vi "Set_Det.vi"(8 "error in (no error)":errorcluster, 11 "Control-Server in":refnum<class "Control-Server.lvclass">) -> (0 "error out":errorcluster, 3 "Control-Server out":refnum<class "Control-Server.lvclass">)   [LabVIEW 2020, in "Control-Server.lvclass"]
uses:
  Control-Server.lvclass
  Config/config_names_def.ctl
  Detector/Emulate/Emulate.lvclass
  C:/Dev/TRANCON/Classes/Detector/Detector.lvclass
  Detector/VIS-IR/VIS-NIR.lvclass
  Detector/UV-VIS/CCD_camera.lvclass
  Detector/DET_BUNCH/Avantes_bunch.lvclass
  Detector/UV-VIS_AVANTES/UV-VIS_AVANTES.lvclass
  dependecies/ControlsVIs/Clusters-def/Message types.ctl
  Message/Message.lvclass
  Message/Message.lvclass/Message.ctl
  GeneralFunctionality/GeneralFunctionality.lvclass/GeneralFunctionality.ctl
  Detector/Detector.lvclass/Detector.ctl
  Control-Server.lvclass/Control-Server.ctl
  Detector/Detector.lvclass
  C:/Dev/TRANCON/Classes/GeneralFunctionality/GeneralFunctionality.lvclass
  Config/Config.lvclass
  GeneralFunctionality/GeneralFunctionality.lvclass
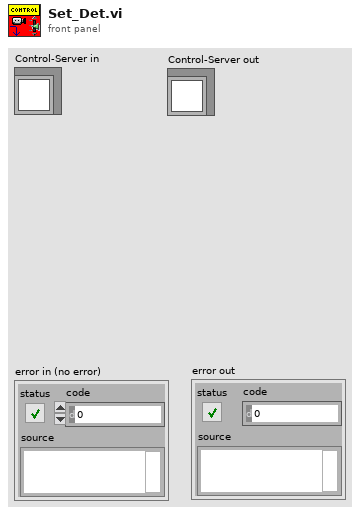
[diagram p1: front panel]
types:
  T1 = typedef "Message types.ctl" = string
  T2 = typedef "Config.lvclass/config_names_def.ctl" = string
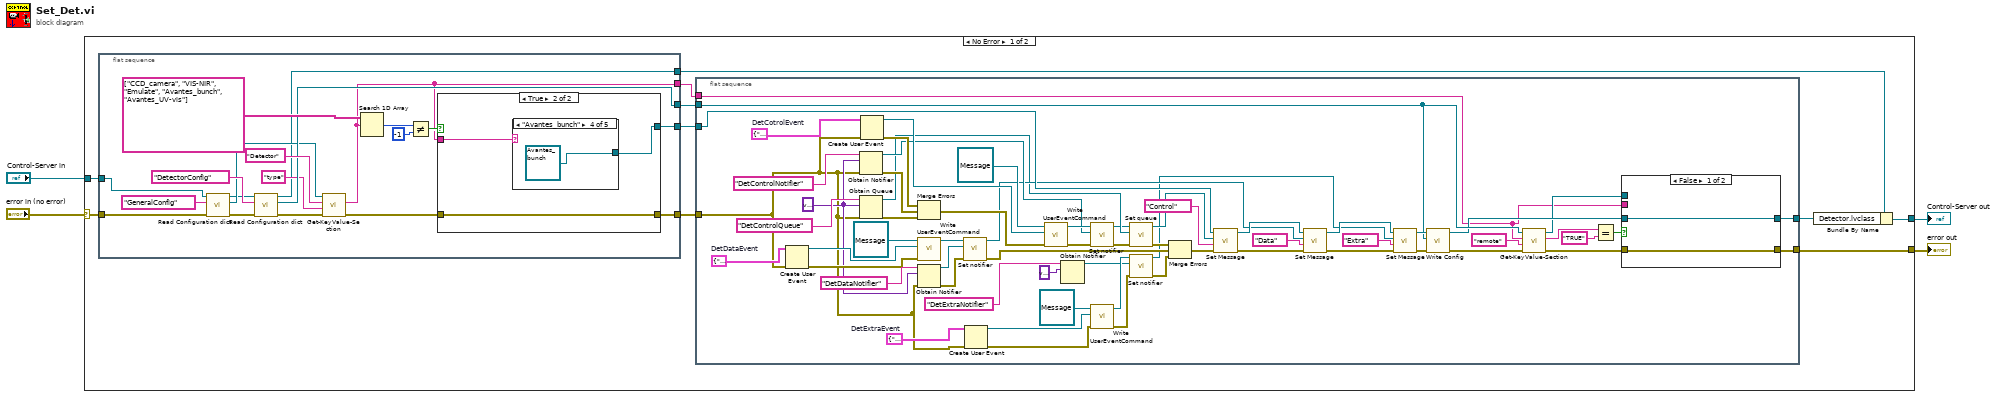
[diagram p0: block diagram]
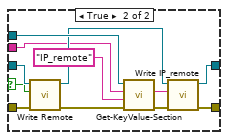
[diagram p2: hidden frame]
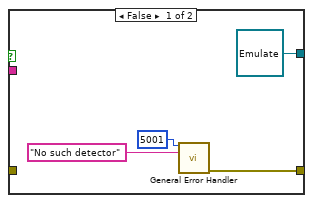
[diagram p3: hidden frame]
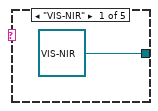
[diagram p4: hidden frame]
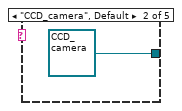
[diagram p5: hidden frame]
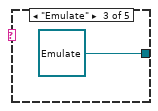
[diagram p6: hidden frame]
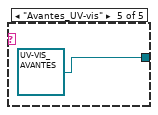
[diagram p7: hidden frame]
diagram:
  n1 = case shown="No Error" "error in (no error)" {
    selector: "error in (no error)" -> [w8 w124]
    tunnel: [w11 w125] -> w4
    tunnel: "Control-Server in" -> [w10 w125]
    tunnel: [w6 w124] -> w2
    frame No Error {
      n2 = flat-sequence {
        tunnel: w10 -> [w101]
        tunnel: w8 -> [w100]
        tunnel: [w103] -> w12
        tunnel: [w93] -> w13
        tunnel: [w102] -> w14
        tunnel: [w94] -> w9
        tunnel: [w92] -> w5
        frame #0 {
          n3 = call "Read Configuration dict.vi"("error in (no error)"=w100, "Config Name"=T2 "GeneralConfig", "Control in"=w101) -> ("error out"=w97:errorcluster, "Config"=w98:refnum<class "Config.lvclass">, "Control out"=w95:refnum<class "Control-Server.lvclass">)  [unwired: 6 in]
          n4 = call "Read Configuration dict.vi"("error in (no error)"=w97, "Config Name"=T2 "DetectorConfig", "Control in"=w95) -> ("error out"=w96:errorcluster, "Config"=w103:refnum<class "Config.lvclass">, "Control out"=w94:refnum<class "Control-Server.lvclass">)  [unwired: 6 in]
          n5 = call-dynamic "Get-KeyValue-Section.vi"("error in (no error)"=w96, "Key"="type", "Section"="Detector", "Config in"=w98) -> ("error out"=w105:errorcluster, "Value"=w92:string)  [unwired: 5 in, 1 out]
          n6 = Search 1D Array(1D array=string[] ["CCD_camera", "VIS-NIR", "Emulate", "Avantes_bunch", "Avantes_UV-vis"], element=w92) -> (index of element=w108:i32)  [unwired: 1 in]
          n7 = Not Equal?(x=w108, y=-1) -> (x != y?=w106:bool)
          n8 = case shown="True" w106 {
            tunnel: w92 -> [_ w118]
            tunnel: [refnum<class "Emulate.lvclass"> refnum ("Emulate.lvclass") w116] -> w102
            tunnel: w105 -> [_ w117]
            tunnel: [w113 w117] -> w93
            frame False {
              n9 = call <vilib>:"General Error Handler.vi"("[error code] (0)"=5001 ("code"), "[error source] (\" \")"="No such detector" ("String to Prepend to source (\"\")")) -> ("error out"=w113:errorcluster)  [unwired: 9 in, 4 out]
            }
            frame True {
              n10 = case shown="\"Avantes_bunch\"" w118 {
                tunnel: [refnum<class "VIS-NIR.lvclass"> refnum ("VIS-IR.lvclass") refnum<class "CCD_camera.lvclass"> refnum ("UV-VIS.lvclass") refnum<class "Emulate.lvclass"> refnum ("DETEmulate.lvclass") refnum<class "Avantes_bunch.lvclass"> refnum ("DET_BUNCH.lvclass") refnum<class "UV-VIS_AVANTES.lvclass"> refnum ("UV-VIS_AVANTES.lvclass")] -> w116
                frame "VIS-NIR" {
                }
                frame "CCD_camera", Default {
                }
                frame "Emulate" {
                }
                frame "Avantes_bunch" {
                }
                frame "Avantes_UV-vis" {
                }
              }
            }
          }
        }
      }
      n11 = flat-sequence {
        tunnel: w12 -> [w25]
        tunnel: w13 -> [w34]
        tunnel: w14 -> [w67]
        tunnel: [w24] -> w7
        tunnel: [w23] -> w6
        tunnel: w5 -> [w18]
        frame #0 {
          w35 = cluster{"command":string, "data":variant} {"command"="", "data"=variant}  # DetExtraEvent
          w44 = variant
          w66 = cluster{"command":string, "data":variant} {"command"="", "data"=variant}  # DetDataEvent
          w73 = cluster{"command":string, "data":variant} {"command"="", "data"=variant}  # DetCotrolEvent
          n12 = Create User Event(user event datatype=w66, error in=w34) -> (user event=w62:refnum<user-event>, error out=w61:errorcluster)
          n13 = Obtain Notifier(name (unnamed)="DetControlNotifier" ("nom (aucun)"), notification data type=w44, error in (no error)=w34) -> (notifier out=w69:refnum<notifier>, error out=w70:errorcluster)  [unwired: 1 in, 1 out]
          n14 = Obtain Queue(name (unnamed)="DetControlQueue", element data type=w44, error in (no error)=w34) -> (queue out=w50:refnum<queue>, error out=w49:errorcluster)  [unwired: 2 in, 1 out]
          n15 = Create User Event(user event datatype=w73, error in=w34) -> (user event=w75:refnum<user-event>, error out=w71:errorcluster)
          n16 = Merge Errors(w71, w70, w49) -> (w68:errorcluster)
          n17 = call "Write UserEventCommand.vi"("error in (no error)"=w61, "UserEventCommand"=w62, "Message en entrée"=refnum<class "Message.lvclass"> refnum ("Message.lvclass")) -> ("Message en sortie"=w63:refnum<class "Message.lvclass">)  [unwired: 7 in, 1 out]
          n18 = Obtain Notifier(name (unnamed)="DetDataNotifier" ("nom (aucun)"), notification data type=w44, error in (no error)=w34) -> (notifier out=w59:refnum<notifier>, error out=w60:errorcluster)  [unwired: 1 in, 1 out]
          n19 = call "Set notifier.vi"("error in (no error)"=w60, "notifier"=w59, "Message en entrée"=w63) -> ("error out"=w58:errorcluster, "Message en sortie"=w54:refnum<class "Message.lvclass">)  [unwired: 7 in]
          n20 = Create User Event(user event datatype=w35, error in=w34) -> (user event=w37:refnum<user-event>, error out=w36:errorcluster)
          n21 = call "Write UserEventCommand.vi"("error in (no error)"=w68, "UserEventCommand"=w75, "Message en entrée"=refnum<class "Message.lvclass"> refnum ("Message.lvclass")) -> ("error out"=w72:errorcluster, "Message en sortie"=w76:refnum<class "Message.lvclass">)  [unwired: 7 in]
          n22 = Obtain Notifier(name (unnamed)="DetExtraNotifier" ("nom (aucun)"), notification data type=variant) -> (notifier out=w29:refnum<notifier>)  [unwired: 2 in, 2 out]
          n23 = call "Set notifier.vi"("error in (no error)"=w72, "notifier"=w69, "Message en entrée"=w76) -> ("error out"=w48:errorcluster, "Message en sortie"=w46:refnum<class "Message.lvclass">)  [unwired: 7 in]
          n24 = call "Write UserEventCommand.vi"("error in (no error)"=w36, "UserEventCommand"=w37, "Message en entrée"=refnum<class "Message.lvclass"> refnum ("Message.lvclass")) -> ("error out"=w32:errorcluster, "Message en sortie"=w33:refnum<class "Message.lvclass">)  [unwired: 7 in]
          n25 = call "Set queue.vi"("error in (no error)"=w48, "queue"=w50, "Message in"=w46) -> ("error out"=w47:errorcluster, "Message out"=w45:refnum<class "Message.lvclass">)  [unwired: 7 in]
          n26 = call "Set notifier.vi"("error in (no error)"=w32, "notifier"=w29, "Message en entrée"=w33) -> ("error out"=w28:errorcluster, "Message en sortie"=w39:refnum<class "Message.lvclass">)  [unwired: 7 in]
          n27 = Merge Errors(w47, w58, w28) -> (w57:errorcluster)
          n28 = call "Set Message.vi"("error in (no error)"=w57, "Message type"=T1 "Control", "Message.lvclass"=w45, "GeneralFunctionality en entrée"=w67) -> ("error out"=w55:errorcluster, "GeneralFunctionality en sortie"=w56:refnum<class "Detector.lvclass">)  [unwired: 6 in]
          n29 = call "Set Message.vi"("error in (no error)"=w55, "Message type"=T1 "Data", "Message.lvclass"=w54, "GeneralFunctionality en entrée"=w56) -> ("error out"=w43:errorcluster, "GeneralFunctionality en sortie"=w40:refnum<class "Detector.lvclass">)  [unwired: 6 in]
          n30 = call "Set Message.vi"("error in (no error)"=w43, "Message type"=T1 "Extra", "Message.lvclass"=w39, "GeneralFunctionality en entrée"=w40) -> ("error out"=w42:errorcluster, "GeneralFunctionality en sortie"=w41:refnum<class "Detector.lvclass">)  [unwired: 6 in]
          n31 = call "Write Config.vi"("error in (no error)"=w42, "Config.lvclass"=w25, "GeneralFunctionality en entrée"=w41) -> ("error out"=w26:errorcluster, "GeneralFunctionality en sortie"=w21:refnum<class "Detector.lvclass">)  [unwired: 7 in]
          n32 = call-dynamic "Get-KeyValue-Section.vi"("error in (no error)"=w26, "Key"="remote", "Section"=w18, "Config in"=w25) -> ("error out"=w22:errorcluster, "Value"=w17:string, "Config out"=w19:refnum<class "Config.lvclass">)  [unwired: 5 in]
          n33 = Equal?(x=w17, y="TRUE") -> (x = y?=w15:bool)
          n34 = case shown="False" w15 {
            selector: w15 -> [_ w80]
            tunnel: [w79 w91] -> w24
            tunnel: [w78 w90] -> w23
            tunnel: w22 -> [w78 w89]
            tunnel: w21 -> [w79 w88]
            tunnel: w19 -> [_ w86]
            tunnel: w18 -> [_ w82]
            frame False {
            }
            frame True {
              n35 = call "Write Remote.vi"("error in (no error)"=w89, "Remote"=w80, "Detector in"=w88) -> ("error out"=w87:errorcluster, "Detector out"=w85:refnum<class "Detector.lvclass">)  [unwired: 7 in]
              n36 = call-dynamic "Get-KeyValue-Section.vi"("error in (no error)"=w87, "Key"="IP_remote", "Section"=w82, "Config in"=w86) -> ("error out"=w83:errorcluster, "Value"=w84:string)  [unwired: 5 in, 1 out]
              n37 = call "Write IP_remote.vi"("error in (no error)"=w83, "IP_remote"=w84, "Detector in"=w85) -> ("error out"=w90:errorcluster, "Detector out"=w91:refnum<class "Detector.lvclass">)  [unwired: 7 in]
            }
          }
        }
      }
      n38 = Bundle By Name(cluster=w9, "Detector.lvclass"=w7) -> (w11:refnum<class "Control-Server.lvclass">)
    }
    frame Error {
    }
  }
  "error out" <- w2
  "Control-Server out" <- w4
